vi "AVQ8347 Ref Level Ref Lebel.vi"(8 "Error In":errorcluster, 9 "Ref Level Unit (dBm)":enum16{"dBm", "mW", "uW", "nW"}(ring), 10 "Ref Level Value (0)":dbl format="%.2f", 11 "VISA Session":refnum<visa-resource-name>) -> (0 "Error Out":errorcluster, 2 "Send Code":string, 3 "Copy VISA Session":refnum<visa-resource-name>)   [LabVIEW 2020]
doc: "Setting of input sensitivity"
panel:
  # "Ref Level Ref Level"
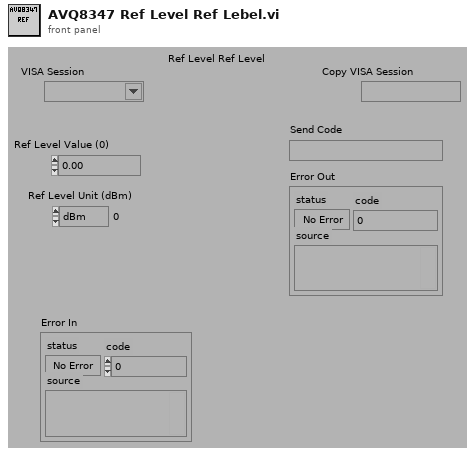
[diagram p1: front panel]
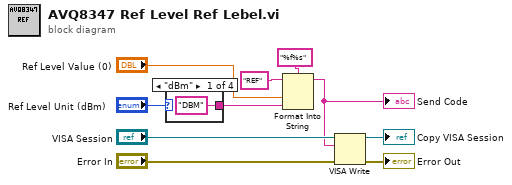
[diagram p0: block diagram]
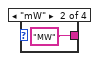
[diagram p2: hidden frame]
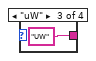
[diagram p3: hidden frame]
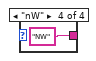
[diagram p4: hidden frame]
diagram:
  n1 = case shown="\"dBm\"" "Ref Level Unit (dBm)" {
    tunnel: ["DBM" "MW" "UW" "NW"] -> w1
    frame "dBm" {
    }
    frame "mW" {
    }
    frame "uW" {
    }
    frame "nW" {
    }
  }
  n2 = Format Into String(format string="%f%s", initial string="REF", "Ref Level Value (0)", w1) -> (resulting string=w2:string)  [unwired: 1 in, 1 out]
  "Send Code" <- w2
  n3 = VISA Write(VISA resource name="VISA Session", write buffer=w2, error in (no error)="Error In") -> (VISA resource name out=→"Copy VISA Session":refnum<visa-resource-name>, error out=→"Error Out":errorcluster)  [unwired: 1 out]
